vi "Ctor.vi"(8 "error in (no error)":errorcluster, 11 "SequenceViewPanel in":refnum<class "SequenceViewPanel.lvclass">) -> (0 "error out":errorcluster, 3 "SequenceViewPanel out":refnum<class "SequenceViewPanel.lvclass">)   [LabVIEW 2020, in "TSnax UI.lvlib" / "SequenceViewPanel.lvclass"]
uses:
  SequenceViewPanel.lvclass
  <vilib>/IlluminatedG/IG OOPanel/OOPanel/Panel/Panel.lvclass
  SequenceViewPanel.lvclass/SequenceViewPanel.ctl
  Ref Data.ctl
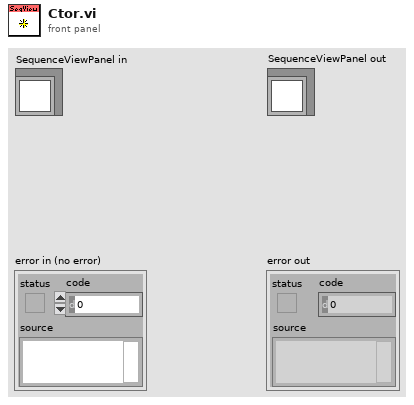
[diagram p1: front panel]
types:
  T1 = typedef "TSnax UI.lvlib/SequenceViewPanel.lvclass/Ref Data.ctl" = cluster{"Insert Index":i32}
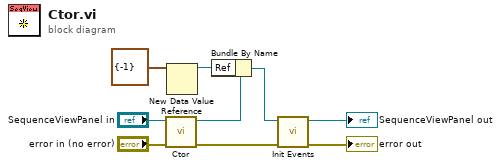
[diagram p0: block diagram]
diagram:
  n1 = call-parent "Ctor.vi"("error in (no error)"="error in (no error)", "Panel in"="SequenceViewPanel in") -> ("error out"=w4:errorcluster, "Panel out"=w6:refnum<class "SequenceViewPanel.lvclass">)  [unwired: 8 in]
  n2 = New Data Value Reference(data value=T1 {"Insert Index"=-1} ("Ref Data")) -> (data value reference=w1:refnum<data-value>)  [unwired: 1 in, 1 out]
  n3 = Bundle By Name(cluster=w6, "Ref"=w1) -> (w2:refnum<class "SequenceViewPanel.lvclass">)
  n4 = call "Init Events.vi"("error in (no error)"=w4, "SequenceViewPanel in"=w2) -> ("error out"=→"error out":errorcluster, "SequenceViewPanel out"=→"SequenceViewPanel out":refnum<class "SequenceViewPanel.lvclass">)  [unwired: 8 in]
